vi "SW_Make_Track_overlay_test.vi"(4 "Pen properties":T1, 5 "Full track array":T2(array[cluster]), 6 "Full trace color":u32(colorbox)=16711680, 7 "Picture in":picture) -> (1 "Picture out":picture)   [LabVIEW 2018, in "Tracker.lvlib"]
uses:
  Tracker.lvlib
panel:
  out "Time to render, s":dbl
  out "Final length":i32 format="%^.0g"
  out "Starting length":i32 format="%^.0g"
  in  "Input colors array":u32[](array[colorbox])=[255, 65535, 6618880, 16776960, 16744448, 16711680]
  out "Colors array":u32[](array[colorbox])
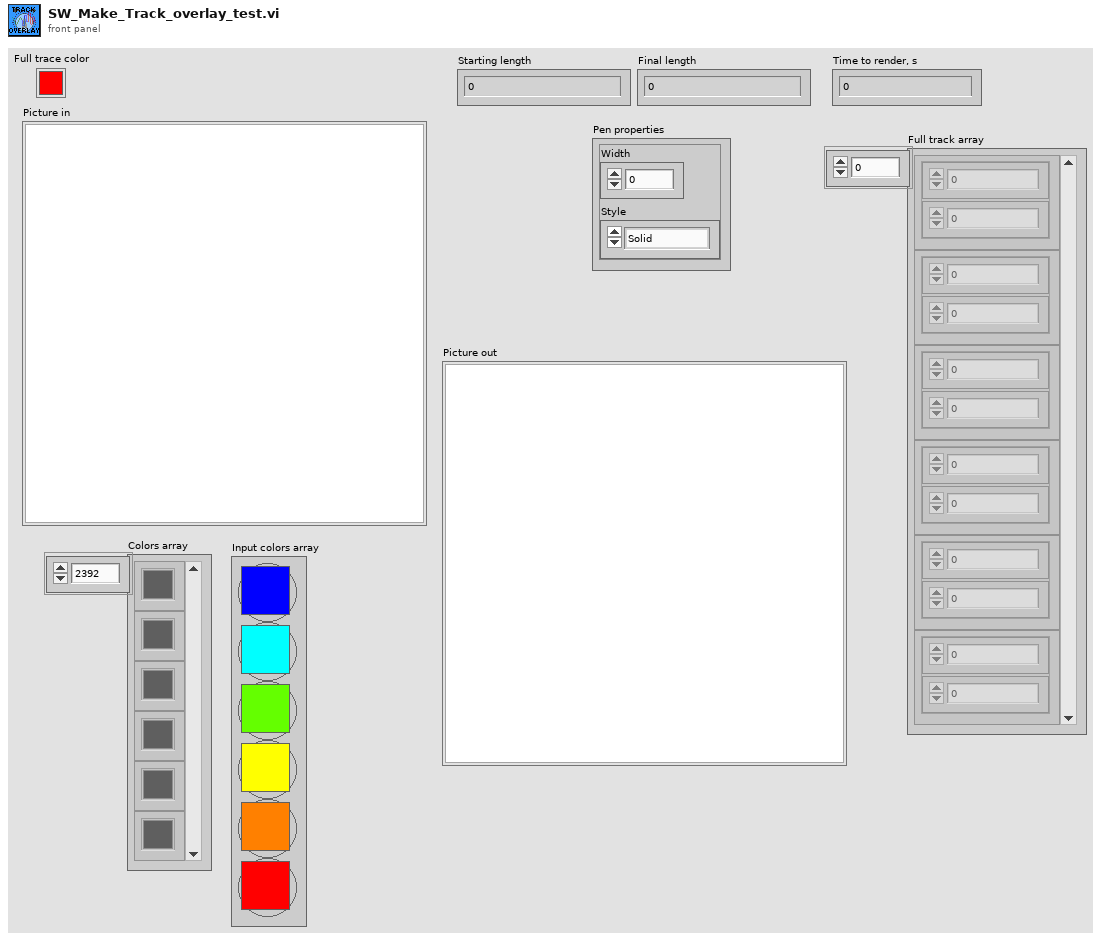
[diagram p1: front panel]
types:
  T1 = cluster{"Width":u16, "Style":enum32{"Solid", "Dash", "Dot", "DashDot", "DashDotDot"}}
  T2 = cluster{"Numeric Control":dbl, "Numeric Control":dbl}[]
  T3 = cluster{"Numeric Control":dbl, "Numeric Control":dbl}
  T4 = cluster{"Numeric Control":i16, "Numeric Control":i16}
  T5 = typedef "imagedata.ctl" = cluster{"image type":i32, "image depth":i32, "image":u8[], "mask":u8[], "colors":u32[], "Rectangle":cluster{"left":i16, "top":i16, "right":i16, "bottom":i16}}
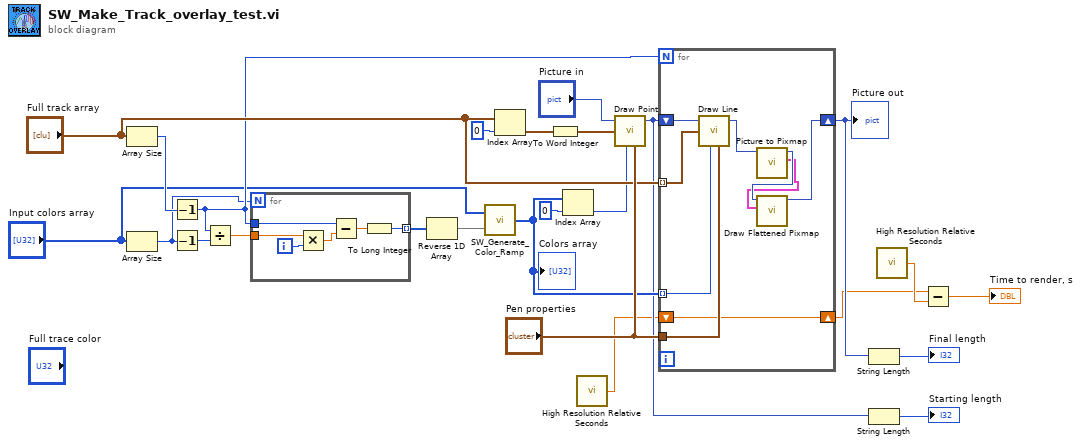
[diagram p0: block diagram]
diagram:
  n1 = Array Size(array="Full track array") -> (size(s)=w19:i32)
  n2 = Array Size(array="Input colors array") -> (size(s)=w12:i32)
  n3 = Decrement(x=w19) -> (x-1=w14:i32)
  n4 = Decrement(x=w12) -> (x-1=w17:i32)
  n5 = Divide(x=w14, y=w17) -> (x/y=w18:dbl)
  n6 = for {
    N: w12 -> [_]
    tunnel: [w26] -> w16 mode=indexing
    tunnel: w14 -> [w31]
    tunnel: w18 -> [w29]
    i -> [w27]
    n7 = Multiply(x=w29, y=w27) -> (x*y=w30:dbl)
    n8 = Subtract(x=w31, y=w30) -> (x-y=w28:dbl)
    n9 = To Long Integer(number=w28) -> (32bit integer=w26:i32)
  }
  n10 = Reverse 1D Array(array=w16) -> (reversed array=w15:i32[])
  n11 = call "SW_Generate_Color_Ramp.vi"("Colors rel. pos."=w15, "Colors array"="Input colors array") -> ("Colors array"=w11:u32[])
  "Colors array" <- w11
  n12 = Index Array(array="Full track array", index=0) -> (element=w23:T3)
  n13 = To Word Integer(number=w23) -> (16bit integer=w21:T4)
  n14 = Index Array(array=w11, index=0) -> (element=w9:u32)
  n15 = call <vilib>:"High Resolution Relative Seconds.vi"() -> ("relative seconds"=w4:dbl)
  n16 = call <vilib>:"Draw Point.vi"("picture"="Picture in", "point(x,y)"=w21, "color(black)"=w9, "pen"="Pen properties") -> ("new picture"=w8:picture)  [unwired: 5 in]
  n17 = for {
    N: w14 -> [_]
    tunnel: "Pen properties" -> [w40]
    shift-right: [w33] -> w6
    shift-left: w8 -> [w38]
    tunnel: "Full track array" -> [w39] mode=indexing
    tunnel: w11 -> [w37] mode=indexing
    shift-right: [w36] -> w2
    shift-left: w4 -> [w36]
    n18 = call <vilib>:"Draw Line.vi"("picture"=w38, "end point"=w39, "color(black)"=w37, "pen"=w40) -> ("new picture"=w35:picture)  [unwired: 5 in]
    n19 = call <vilib>:"Picture to Pixmap.vi"("picture"=w35) -> ("image data"=w32:T5, "new picture"=w34:picture)  [unwired: 9 in]
    n20 = call <vilib>:"Draw Flattened Pixmap.vi"("image data"=w32, "picture"=w34) -> ("new picture"=w33:picture)  [unwired: 7 in]
  }
  "Picture out" <- w6
  n21 = String Length(string=w6) -> (length=→"Final length":i32)
  n22 = String Length(string=w8) -> (length=→"Starting length":i32)
  n23 = call <vilib>:"High Resolution Relative Seconds.vi"() -> ("relative seconds"=w3:dbl)
  n24 = Subtract(x=w2, y=w3) -> (x-y=→"Time to render, s":dbl)
